vi "IsRepeatTag__slk_mt.vi"(8 "error in (no error)":errorcluster, 10 "tag":string, 11 "tree view in":refnum<class "TreeView__slk_mt.lvclass">) -> (0 "error out":errorcluster, 2 "repeat?":bool, 3 "tree view out":refnum<class "TreeView__slk_mt.lvclass">)   [LabVIEW 2012, in "Lazyboots Menu Tool.lvlib" / "TreeView__slk_mt.lvclass"]
doc: "Checks if the tag is repeated."
uses:
  TreeView__slk_mt.lvclass
panel:
  # "IsRepeatTag__slk_mt.vi\nChecks if the tag is repeated.\n\nNOTICE -- YOU MUST LEAVE THIS NOTICE IN PLACE.\n\nCopyright (c) 2011, LIANG LIU Shawn.Liu.cn@gmail.com\nAll rights reserved.\n\nRedistribution and use in source and binary forms, with or without modification, are permitted provided that the following conditions are met:\n-Redistributions of source code must retain the above copyright notice, this list of conditions and the following disclaimer.\n-Redistributions in binary form must reproduce the above copyright notice, this list of conditions and the following disclaimer in the documentation and/or other materials provided with the distribution.\n-Neither the name of the eLp nor the names of its contributors may be used to endorse or promote products derived from this software without specific prior written permission.\n\nTHIS SOFTWARE IS PROVIDED BY THE COPYRIGHT HOLDERS AND CONTRIBUTORS \"AS IS\" AND ANY EXPRESS OR IMPLIED WARRANTIES, INCLUDING, BUT NOT LIMITED TO, THE IMPLIED WARRANTIES OF MERCHANTABILITY AND FITNESS FOR A PARTICULAR PURPOSE ARE DISCLAIMED. IN NO EVENT SHALL THE COPYRIGHT HOLDER OR CONTRIBUTORS BE LIABLE FOR ANY DIRECT, INDIRECT, INCIDENTAL, SPECIAL, EXEMPLARY, OR CONSEQUENTIAL DAMAGES (INCLUDING, BUT NOT LIMITED TO, PROCUREMENT OF SUBSTITUTE GOODS OR SERVICES; LOSS OF USE, DATA, OR PROFITS; OR BUSINESS INTERRUPTION) HOWEVER CAUSED AND ON ANY THEORY OF LIABILITY, WHETHER IN CONTRACT, STRICT LIABILITY, OR TORT (INCLUDING NEGLIGENCE OR OTHERWISE) ARISING IN ANY WAY OUT OF THE USE OF THIS SOFTWARE, EVEN IF ADVISED OF THE POSSIBILITY OF SUCH DAMAGE."
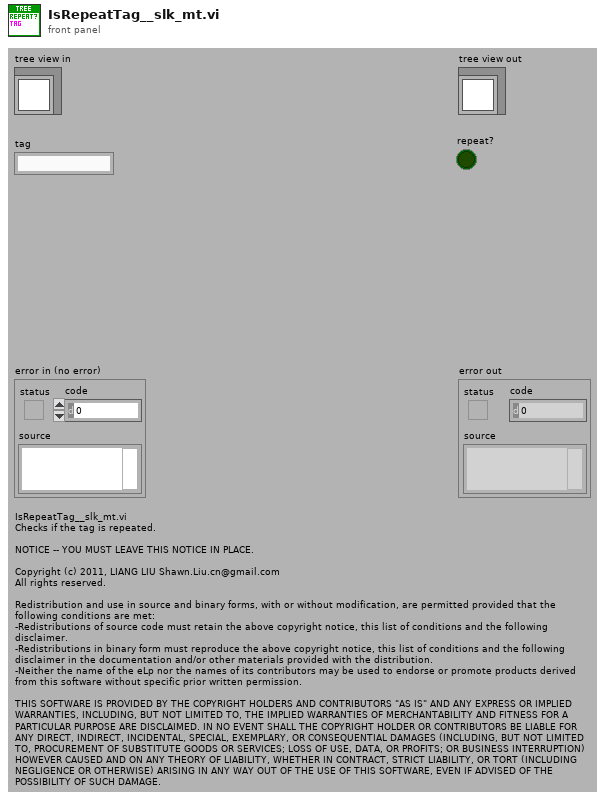
[diagram p1: front panel]
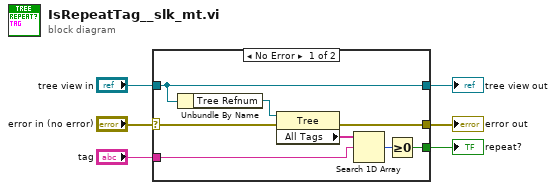
[diagram p0: block diagram]
diagram:
  n1 = case shown="No Error" "error in (no error)" {
    selector: "error in (no error)" -> [w8 w16]
    tunnel: [w11 w16] -> w5
    tunnel: [w14 w15] -> w3
    tunnel: "tree view in" -> [w14 w15]
    tunnel: "tag" -> [w7 _]
    tunnel: [w9 _] -> w2
    frame No Error {
      n2 = Unbundle By Name(w14) -> ("Tree Refnum"=w13:refnum<vi>)
      n3 = property class="Tree"(reference=w13, error in=w8) -> (error out=w11:errorcluster, "All Tags"=w12:string[])  [unwired: 1 out]
      n4 = Search 1D Array(1D array=w12, element=w7) -> (index of element=w10:i32)  [unwired: 1 in]
      n5 = Greater Or Equal To 0?(x=w10) -> (x >= 0?=w9:bool)
    }
    frame Error {
    }
  }
  "error out" <- w5
  "tree view out" <- w3
  "repeat?" <- w2
